vi "TestVI.vi"   [LabVIEW 2017]
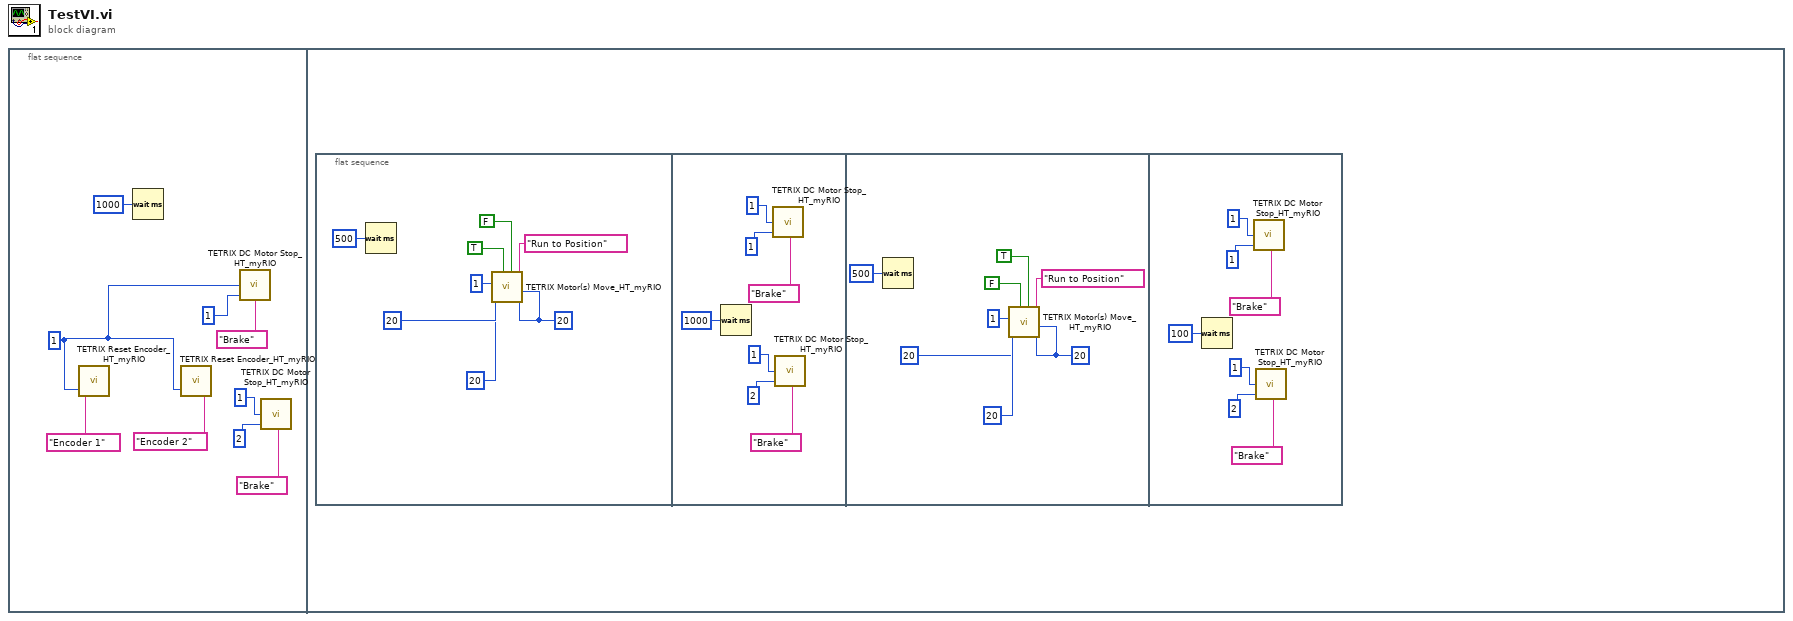
[diagram p0: block diagram]
diagram:
  n1 = flat-sequence {
    frame #0 {
      w3 = u8 1 ("Controller Daisy Chain Position ( 1 - 4)")
      n2 = call <vilib>:"TETRIX Reset Encoder_HT_myRIO.vi"("Select Encoder"="Encoder 1", "Controller Daisy Chain Position ( 1 - 4)"=w3) -> ()  [unwired: 1 in, 1 out]
      n3 = Wait (ms)(milliseconds to wait=u32 1000) -> ()  [unwired: 1 out]
      n4 = call <vilib>:"TETRIX Reset Encoder_HT_myRIO.vi"("Select Encoder"="Encoder 2", "Controller Daisy Chain Position ( 1 - 4)"=w3) -> ()  [unwired: 1 in, 1 out]
      n5 = call <vilib>:"TETRIX DC Motor Stop_HT_myRIO.vi"("Stop (Brake or Coast)"="Brake", "Motor Channel: (1 or 2)"=u8 1, "Controller Daisy Chain Position: 1 - 4"=w3) -> ()  [unwired: 1 in, 1 out]
      n6 = call <vilib>:"TETRIX DC Motor Stop_HT_myRIO.vi"("Stop (Brake or Coast)"="Brake", "Motor Channel: (1 or 2)"=u8 2, "Controller Daisy Chain Position: 1 - 4"=u8 1) -> ()  [unwired: 1 in, 1 out]
    }
    frame #1 {
      n7 = flat-sequence {
        frame #0 {
          w14 = i8 20 ("Motor 2 Power (-100 to 100)\n0 = Stop/Brake\n-128 = Stop/Coast")
          n8 = Wait (ms)(milliseconds to wait=u32 500) -> ()  [unwired: 1 out]
          n9 = call <vilib>:"TETRIX Motor(s) Move_HT_myRIO.vi"("Motor 2 Power (-100 to 100)\n0 = Stop/Brake\n-128 = Stop/Coast"=w14, "Motor 1 Power (-100 to 100)\n0 = Stop/Brake\n-128 = Stop/Coast"=w14, "Control Mode"="Run to Position", "Motor 2 Reverse? : T or F"=FALSE, "Motor 1 Reverse? : T or F"=TRUE, "Encoder 2 Target: 360 = 1 motor shaft revolution"=20, "Encoder 1 Target: 360 = 1 motor shaft revolution"=20, "Controller Daisy Chain Position: 1 - 4"=u8 1) -> ()  [unwired: 1 in, 1 out]
        }
        frame #1 {
          n10 = Wait (ms)(milliseconds to wait=u32 1000) -> ()  [unwired: 1 out]
          n11 = call <vilib>:"TETRIX DC Motor Stop_HT_myRIO.vi"("Stop (Brake or Coast)"="Brake", "Motor Channel: (1 or 2)"=u8 1, "Controller Daisy Chain Position: 1 - 4"=u8 1) -> ()  [unwired: 1 in, 1 out]
          n12 = call <vilib>:"TETRIX DC Motor Stop_HT_myRIO.vi"("Stop (Brake or Coast)"="Brake", "Motor Channel: (1 or 2)"=u8 2, "Controller Daisy Chain Position: 1 - 4"=u8 1) -> ()  [unwired: 1 in, 1 out]
        }
        frame #2 {
          w28 = i8 20 ("Motor 2 Power (-100 to 100)\n0 = Stop/Brake\n-128 = Stop/Coast")
          n13 = Wait (ms)(milliseconds to wait=u32 500) -> ()  [unwired: 1 out]
          n14 = call <vilib>:"TETRIX Motor(s) Move_HT_myRIO.vi"("Motor 2 Power (-100 to 100)\n0 = Stop/Brake\n-128 = Stop/Coast"=w28, "Motor 1 Power (-100 to 100)\n0 = Stop/Brake\n-128 = Stop/Coast"=w28, "Control Mode"="Run to Position", "Motor 2 Reverse? : T or F"=TRUE, "Motor 1 Reverse? : T or F"=FALSE, "Encoder 2 Target: 360 = 1 motor shaft revolution"=20, "Encoder 1 Target: 360 = 1 motor shaft revolution"=20, "Controller Daisy Chain Position: 1 - 4"=u8 1) -> ()  [unwired: 1 in, 1 out]
        }
        frame #3 {
          n15 = Wait (ms)(milliseconds to wait=u32 100) -> ()  [unwired: 1 out]
          n16 = call <vilib>:"TETRIX DC Motor Stop_HT_myRIO.vi"("Stop (Brake or Coast)"="Brake", "Motor Channel: (1 or 2)"=u8 1, "Controller Daisy Chain Position: 1 - 4"=u8 1) -> ()  [unwired: 1 in, 1 out]
          n17 = call <vilib>:"TETRIX DC Motor Stop_HT_myRIO.vi"("Stop (Brake or Coast)"="Brake", "Motor Channel: (1 or 2)"=u8 2, "Controller Daisy Chain Position: 1 - 4"=u8 1) -> ()  [unwired: 1 in, 1 out]
        }
      }
    }
  }
